vi "zad1.vi"() -> ()   [LabVIEW 2017]
uses:
  <vilib>/measure/NI_MABase.lvlib
panel:
  out "output":dbl
  in  "input":dbl
  in  "frequency":dbl=10.0 format="%0.2p"
  out "Waveform Graph 2":waveform(dbl)(graph)
  out "Waveform Graph":waveform(dbl)(graph)
  in  "stop":bool
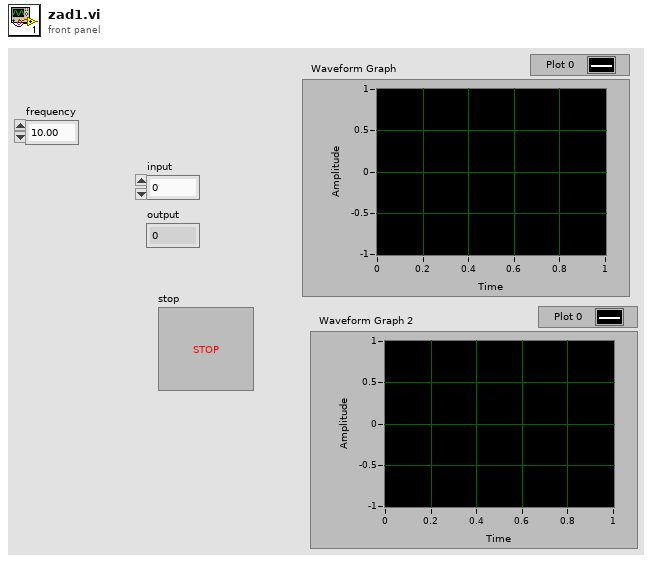
[diagram p1: front panel]
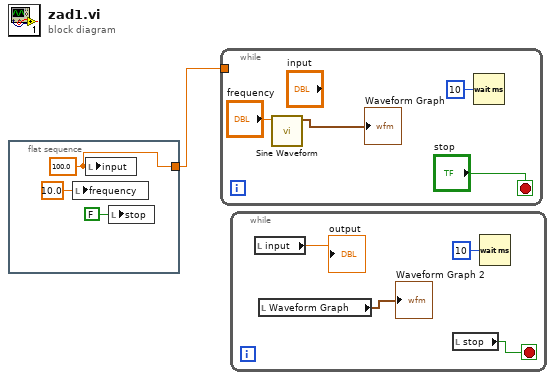
[diagram p0: block diagram]
diagram:
  n1 = flat-sequence {
    tunnel: [w2] -> w1
    frame #0 {
      w2 = 100.0 ("input")
      n2 = local write "frequency"(10.0 ("frequency")) -> ()
      n3 = local write "input"(w2) -> ()
      n4 = local write "stop"(FALSE ("stop")) -> ()
    }
  }
  n5 = while {
    tunnel: w1 -> [_]
    stop <- "stop" stop-if-true
    n6 = call <vilib>:"Sine Waveform.vi"("frequency"="frequency") -> ("signal out"=→"Waveform Graph":waveform(dbl))  [unwired: 9 in, 1 out]
    n7 = Wait (ms)(milliseconds to wait=u32 10) -> ()  [unwired: 1 out]
  }
  n8 = while {
    stop <- w12 stop-if-true
    n9 = local read "input"() -> (→"output":dbl)
    n10 = local read "Waveform Graph"() -> (→"Waveform Graph 2":waveform(dbl))
    n11 = local read "stop"() -> (w12:bool)
    n12 = Wait (ms)(milliseconds to wait=u32 10) -> ()  [unwired: 1 out]
  }
